vi "2 - QDSM state as class.vi"() -> ()   [LabVIEW 2015]
uses:
  State/Parent Actor.lvclass
  Child Actor/Child Actor.lvclass
panel:
  in  "Choose Actor":bool
  out "On Off Indicator":bool
  out "Dirrection indicator":enum16{"Forward", "Reverse"}(ring)
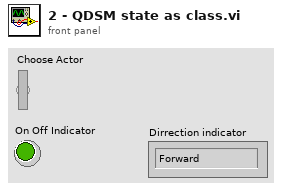
[diagram p1: front panel]
types:
  T1 = cluster{"Command":string, "Data":enum16{"Forward", "Reverse"}}
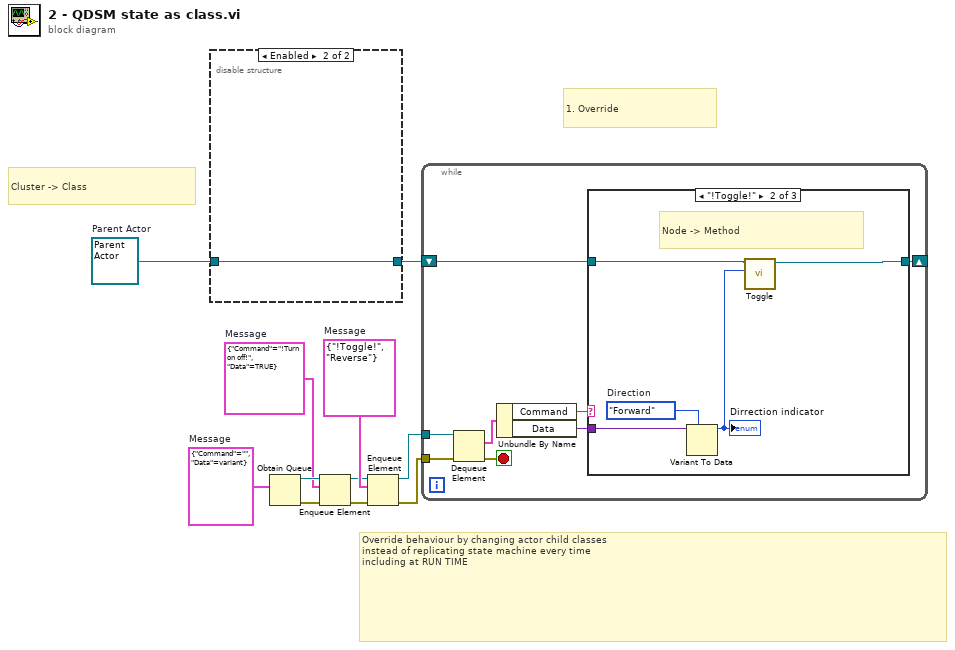
[diagram p0: block diagram]
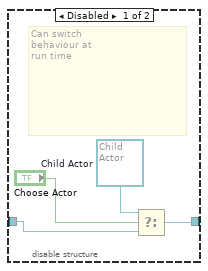
[diagram p2: hidden frame]
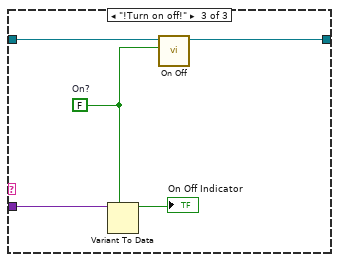
[diagram p4: hidden frame]
diagram:
  w2 = refnum<class "Parent Actor.lvclass"> refnum  # Parent Actor
  w3 = cluster{"Command":string, "Data":bool} {"Command"="!Turn on off!", "Data"=TRUE}  # Message
  w10 = T1 {"Command"="!Toggle!", "Data"=enum."Reverse"}  # Message
  w11 = cluster{"Command":string, "Data":variant} {"Command"="", "Data"=variant}  # Message
  # "1. Override"
  # "Override behaviour by changing actor child classes\ninstead of replicating state machine every time \nincluding at RUN TIME"
  # "Cluster -> Class"
  n1 = disable-structure shown="Enabled" {
    disable-tunnel: w2 -> [w15 w16]
    disable-tunnel: [w13 w16] -> w1
    frame Disabled {
      w14 = refnum<class "Child Actor.lvclass"> refnum  # Child Actor
      # "Can switch \nbehaviour at \nrun time"
      n2 = Select(t=w14, s="Choose Actor", f=w15) -> (s? t:f=w13:refnum<class "Parent Actor.lvclass">)
    }
    frame Enabled {
    }
  }
  n3 = Obtain Queue(element data type=w11) -> (queue out=w5:refnum<queue>, error out=w7:errorcluster)  [unwired: 4 in, 1 out]
  n4 = Enqueue Element(queue=w5, element=w3, error in (no error)=w7) -> (queue out=w4:refnum<queue>, error out=w6:errorcluster)  [unwired: 1 in, 1 out]
  n5 = Enqueue Element(queue=w4, element=w10, error in (no error)=w6) -> (queue out=w8:refnum<queue>, error out=w9:errorcluster)  [unwired: 1 in, 1 out]
  n6 = while {
    tunnel: w9 -> [w24]
    tunnel: w8 -> [w23]
    shift-right: [w17] -> _
    shift-left: w1 -> [w18]
    stop <- w21 stop-if-true
    n7 = Dequeue Element(queue=w23, error in (no error)=w24) -> (element=w22:cluster{"Command":string, "Data":variant}, error out=w21:errorcluster)  [unwired: 1 in, 2 out]
    n8 = Unbundle By Name(w22) -> ("Command"=w20:string, "Data"=w19:variant)
    n9 = case shown="\"!Toggle!\"" w20 {
      tunnel: w19 -> [_ w30 w35]
      tunnel: w18 -> [w25 w27 w34]
      tunnel: [w25 w26 w33] -> w17
      frame "", Default {
      }
      frame "!Toggle!" {
        w29 = enum16{"Forward", "Reverse"}."Forward"  # Direction
        # "Node -> Method"
        n10 = Variant To Data(type=w29, Variant=w30) -> (data=w28:enum16{"Forward", "Reverse"})  [unwired: 1 in, 1 out]
        "Dirrection indicator" <- w28
        n11 = call-dynamic "Toggle.vi"("Dirrection"=w28, "State in"=w27) -> ("State out"=w26:refnum<class "Parent Actor.lvclass">)  [unwired: 8 in, 1 out]
      }
      frame "!Turn on off!" {
        w31 = FALSE  # On?
        n12 = Variant To Data(type=w31, Variant=w35) -> (data=→"On Off Indicator":bool)  [unwired: 1 in, 1 out]
        n13 = call-dynamic "On Off.vi"("On Off"=w31, "State in"=w34) -> ("State out"=w33:refnum<class "Parent Actor.lvclass">)  [unwired: 8 in, 1 out]
      }
    }
  }
